vi "EstadisticaDataReadingStringToClusterFormar.vi"(11 "StringFormat":string[](array[string])) -> (3 "ClusterFormat":T1)   [LabVIEW 2014]
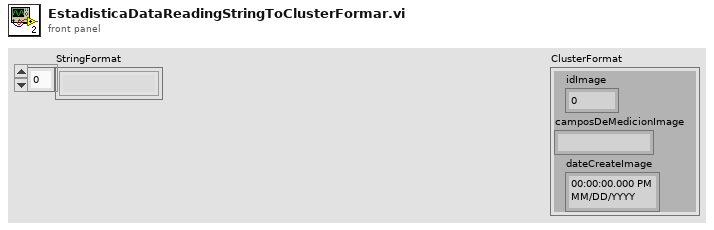
[diagram p1: front panel]
types:
  T1 = cluster{"idImage":dbl, "camposDeMedicionImage":string, "dateCreateImage":timestamp}
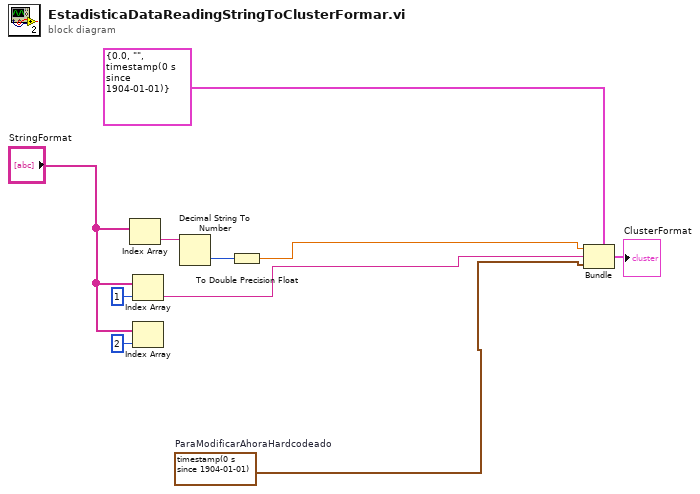
[diagram p0: block diagram]
diagram:
  w2 = timestamp(0 s since 1904-01-01)  # ParaModificarAhoraHardcodeado
  n1 = Index Array(array="StringFormat") -> (element=w10:string)  [unwired: 1 in]
  n2 = Index Array(array="StringFormat", index=1) -> (element=w5:string)
  n3 = Index Array(array="StringFormat", index=2) -> ()  [unwired: 1 out]
  n4 = Decimal String To Number(string=w10) -> (number=w7:i32)  [unwired: 2 in, 1 out]
  n5 = To Double Precision Float(number=w7) -> (double precision float=w6:dbl)
  n6 = Bundle(cluster=T1 {"idImage"=0.0, "camposDeMedicionImage"="", "dateCreateImage"=timestamp(0 s since 1904-01-01)} ("dataToQueryOfRead"), "idImage"=w6, "camposDeMedicionImage"=w5, "dateCreateImage"=w2) -> (→"ClusterFormat":T1)
